vi "Select Test.vi"(11 "Thread in":T3) -> (0 "Skip Test":bool, 1 "Aktív?":bool, 2 "Current Test":T1, 3 "Thread out":T3)   [LabVIEW 2014]
uses:
  Thread.ctl
  Teszt/Teszt.ctl
  Teszt/Command.ctl
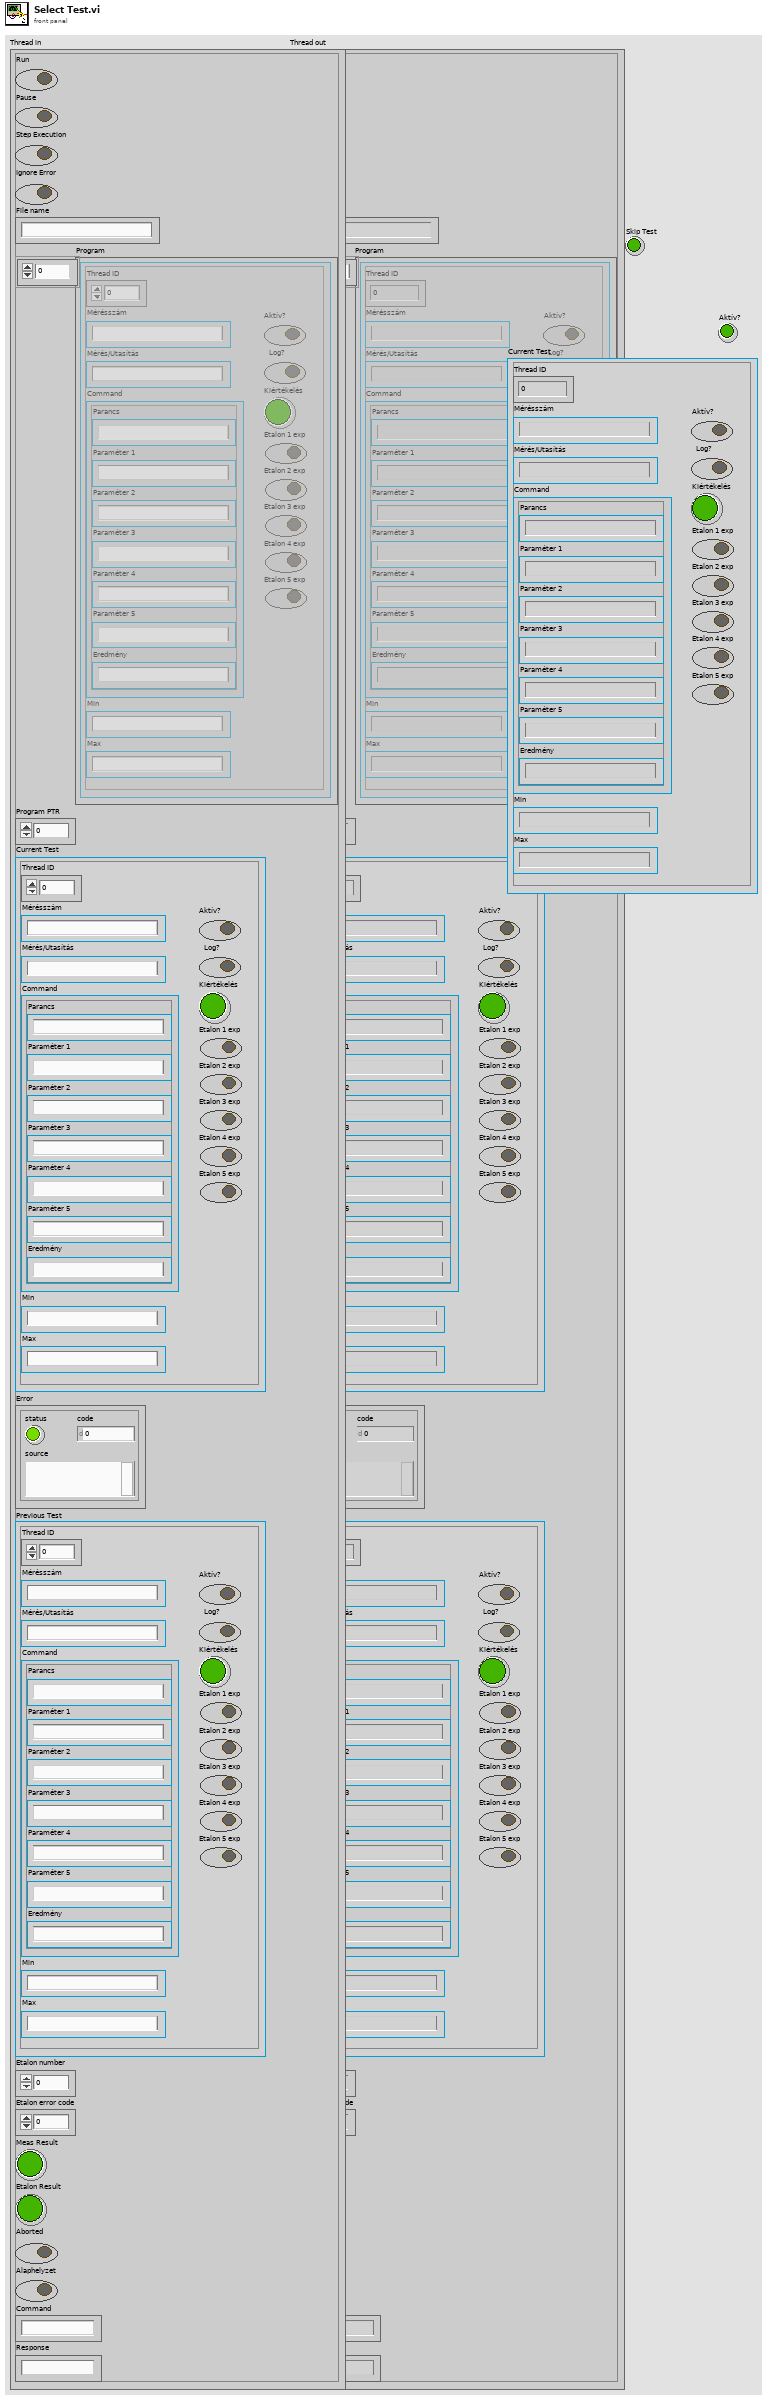
[diagram p1: front panel]
types:
  T1 = typedef "Teszt.ctl" = cluster{"Thread ID":dbl, "Mérésszám":string, "Mérés/Utasítás":string, "Command":T2, "Min":string, "Max":string, "Aktív?":bool, "Log?":bool, "Kiértékelés":bool, "Etalon 1 exp":bool, "Etalon 2 exp":bool, "Etalon 3 exp":bool, "Etalon 4 exp":bool, "Etalon 5 exp":bool}
  T2 = typedef "Command.ctl" = cluster{"Parancs":string, "Paraméter 1":string, "Paraméter 2":string, "Paraméter 3":string, "Paraméter 4":string, "Paraméter 5":string, "Eredmény":string}
  T3 = typedef "Thread.ctl" = cluster{"Run":bool, "Pause":bool, "Step Execution":bool, "Ignore Error":bool, "File name":string, "Program":T1[], "Program PTR":u32, "Current Test":T1, "Error":errorcluster, "Previous Test":T1, "Etalon number":u32, "Etalon error code":u32, "Meas Result":bool, "Etalon Result":bool, "Aborted":bool, "Alaphelyzet":bool, "Command":string, "Response":string}
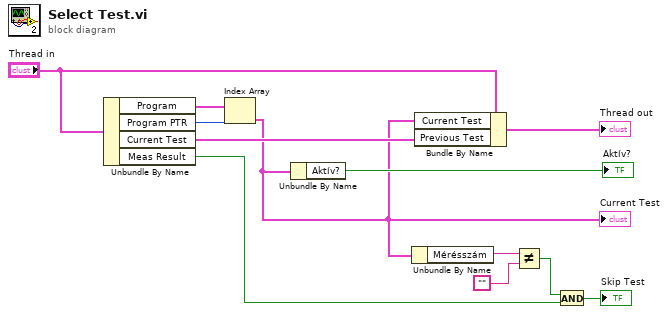
[diagram p0: block diagram]
diagram:
  n1 = Unbundle By Name("Thread in") -> ("Program"=w11:T1[], "Program PTR"=w10:u32, "Current Test"=w8:T1, "Meas Result"=w2:bool)
  n2 = Index Array(array=w11, index=w10) -> (element=w6:T1)
  "Current Test" <- w6
  n3 = Unbundle By Name(w6) -> ("Aktív?"=→"Aktív?":bool)
  n4 = Unbundle By Name(w6) -> ("Mérésszám"=w5:string)
  n5 = Bundle By Name(cluster="Thread in", "Current Test"=w6, "Previous Test"=w8) -> (→"Thread out":T3)
  n6 = Not Equal?(x=w5, y="") -> (x != y?=w3:bool)
  n7 = And(x=w3, y=w2) -> (x .and. y?=→"Skip Test":bool)
